vi "Format+Name (SubVI).vi"(0 "Format+Namen Eingang":string) -> (10 "Trennzeichen":string, 12 "Format-String":string, 14 "Format-ende":string, 16 "Format-Zusatzinformation":string, 20 "1":string, 21 "2":string, 22 "3":string, 23 "4":string, 24 "5":string, 25 "6":string, 26 "7":string, 27 "8":string)   [LabVIEW 2010]
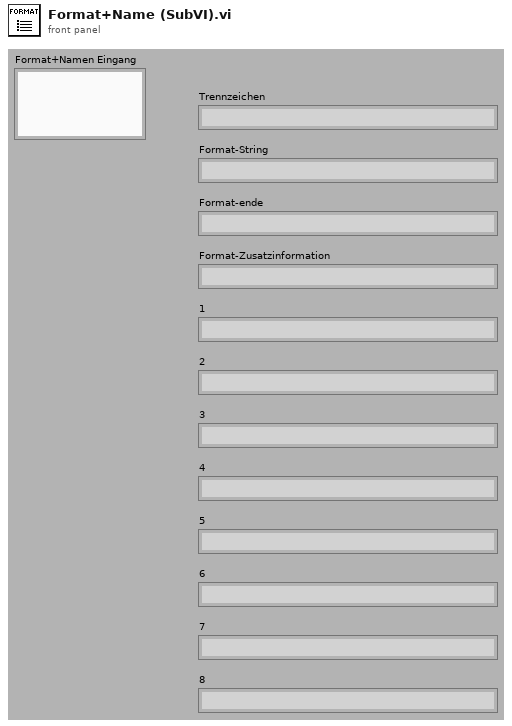
[diagram p1: front panel]
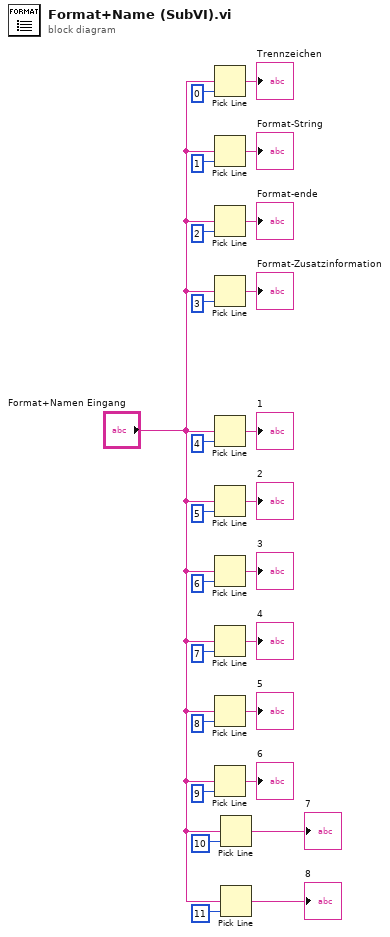
[diagram p0: block diagram]
diagram:
  n1 = Pick Line(multi-line string="Format+Namen Eingang", line index=0 ("Zeilenindex")) -> (output string=→"Trennzeichen":string)  [unwired: 1 in]
  n2 = Pick Line(multi-line string="Format+Namen Eingang", line index=1 ("Zeilenindex")) -> (output string=→"Format-String":string)  [unwired: 1 in]
  n3 = Pick Line(multi-line string="Format+Namen Eingang", line index=2 ("Zeilenindex")) -> (output string=→"Format-ende":string)  [unwired: 1 in]
  n4 = Pick Line(multi-line string="Format+Namen Eingang", line index=3 ("Zeilenindex")) -> (output string=→"Format-Zusatzinformation":string)  [unwired: 1 in]
  n5 = Pick Line(multi-line string="Format+Namen Eingang", line index=4 ("Zeilenindex")) -> (output string=→"1":string)  [unwired: 1 in]
  n6 = Pick Line(multi-line string="Format+Namen Eingang", line index=5 ("Zeilenindex")) -> (output string=→"2":string)  [unwired: 1 in]
  n7 = Pick Line(multi-line string="Format+Namen Eingang", line index=6 ("Zeilenindex")) -> (output string=→"3":string)  [unwired: 1 in]
  n8 = Pick Line(multi-line string="Format+Namen Eingang", line index=7 ("Zeilenindex")) -> (output string=→"4":string)  [unwired: 1 in]
  n9 = Pick Line(multi-line string="Format+Namen Eingang", line index=8 ("Zeilenindex")) -> (output string=→"5":string)  [unwired: 1 in]
  n10 = Pick Line(multi-line string="Format+Namen Eingang", line index=9 ("Zeilenindex")) -> (output string=→"6":string)  [unwired: 1 in]
  n11 = Pick Line(multi-line string="Format+Namen Eingang", line index=10 ("Zeilenindex")) -> (output string=→"7":string)  [unwired: 1 in]
  n12 = Pick Line(multi-line string="Format+Namen Eingang", line index=11 ("Zeilenindex")) -> (output string=→"8":string)  [unwired: 1 in]
